vi "ScriptTest.vi"() -> ()   [LabVIEW 2012]
panel:
  out "Variables":string="0: VER = 9\r\n1: HI = 1\r\n2: LO = 0\r\n3: END = 22\r\n4: variable = 13\r\n5: count1 = 4\r\n6: var = 2\r\n7: array_SIZE = 10\r\n8: array_0 = 0\r\n9: array_1 = 0\r\n10: array_2 = 0\r\n11: array_3 = 3\r\n12: array_4 = 0\r\n13: array_5 = 1\r\n14: array_6 = 0\r\n15: array_7 = 0\r\n16: array_8 = 0\r\n17: array_9 = 0\r\n18: count0 = 2\r\n"
  out "Array":bool[](array[boolean])=[TRUE, TRUE, TRUE, FALSE, TRUE, TRUE, TRUE]
  out "Received replies":string[](array[string])=["0\n1\n2\n4", "1\n1\n1\n1\n1", "1\n50\n1\n1", "1\n0\n200\n231\n247\n1\n200\n226", "10\n1\n0\n3\n3\n3\n0", "[1,115]  start script\n [5,61,0,18,0,0]  \n [5,61,202,13,0,1]  \n [3,87,3,232]  \n [5,61,202,13,0,0]  \n [3,87,3,232]  \n [5,43,0,18,0,1]  \n [8,73,60,255,18,0,2,0,5]  \n [1,101]  \n [1,69]  61,0,18,0,0,61,202,13,0,1,87,3,232,61,202,13,0,0,87,3,232,43,0,18,0,1,73,60,255,18,0,2,0,5,101,end script\n0\n1\n1000\n0\n1000\n1\n5\n1\n1000\n0\n1000\n2\n34\nDone", "2\n [1,115]  start script\n [5,61,202,13,0,0]  \n [8,33,6,255,4,0,13,0,2]  \n [3,119,0,1]  \n [5,61,202,13,0,1]  \n [1,101]  \n [1,69]  61,202,13,0,0,33,6,255,4,0,13,0,2,119,0,1,61,202,13,0,1,101,end script\n0\n13\n1\n1\nDone"]
  in  "Expected replies":string[](array[string])=["0\n1\n2\n4", "1\n1\n1\n1\n1", "1\n50\n1\n1", "1\r\n0\r\n200\r\n226\r\n241\r\n1\r\n200\r\n231\r", "10\n1\n0\n3\n3\n3\n0", "[1,115]  start script\n [5,61,0,18,0,0]  \n [5,61,202,13,0,1]  \n [3,87,3,232]  \n [5,61,202,13,0,0]  \n [3,87,3,232]  \n [5,43,0,18,0,1]  \n [8,73,60,255,18,0,2,0,5]  \n [1,101]  \n [1,69]  61,0,18,0,0,61,202,13,0,1,87,3,232,61,202,13,0,0,87,3,232,43,0,18,0,1,73,60,255,18,0,2,0,5,101,end script\n0\n1\n1000\n0\n1000\n1\n5\n1\n1000\n0\n1000\n2\n34\nDone", "2\n [1,115]  start script\n [5,61,202,13,0,0]  \n [8,33,6,255,4,0,13,0,2]  \n [3,119,0,1]  \n [5,61,202,13,0,1]  \n [1,101]  \n [1,69]  61,202,13,0,0,33,6,255,4,0,13,0,2,119,0,1,61,202,13,0,1,101,end script\n0\n13\n1\n1\nDone"]
  in  "Test codes":string[](array[string])=["SET count1,0\nADD count1,1\nADD count1,count1\nADD count1,count1\n", "SET var,1\nSET DIO[0],1\nSET DIO[2],var\nSET DIO[var],var\nSET DIO[30],1\n", "SET var,1\nSET PWM[0],50\nSET PWM[2],var\nSET PWM[var],var\n", "SET var,1\nSET TMR[1],0\nWAIT 0.2\nGET TMR[1]\nGET TMR[var]\nSET TMR[var],var\nWAIT 0.2\nGET TMR[var]", "SET array_SIZE,10\nSET array[5],1\nGET array[0]\nSET var,3\nSET array[var],var\nGET array[var]\nGET array[10]\n", "SCRIPT\ncount0=0\n//while0 for 2 iterations\nwhileLand0:\nDIO[13] = 1\nWAIT 1.000000\nDIO[13] = 0\nWAIT 1.000000\n//end while0 \ncount0+=1\nIF (count0 < 2) GOTO whileLand0\nend\nENDSCRIPT\nRUN&WAIT 0", "SYSTEM var,2,5\nSCRIPT\nDIO[13] = 0\nSYSTEM variable,13,2\nWAITµs 1.000000\nDIO[13] = 1\nend\nENDSCRIPT\nRUN&WAIT 0"]
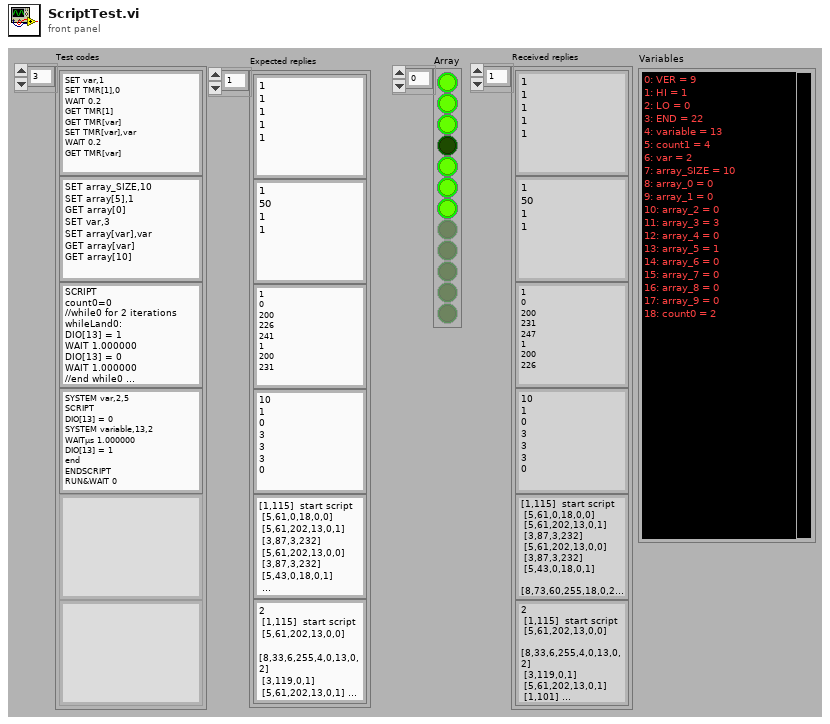
[diagram p1: front panel]
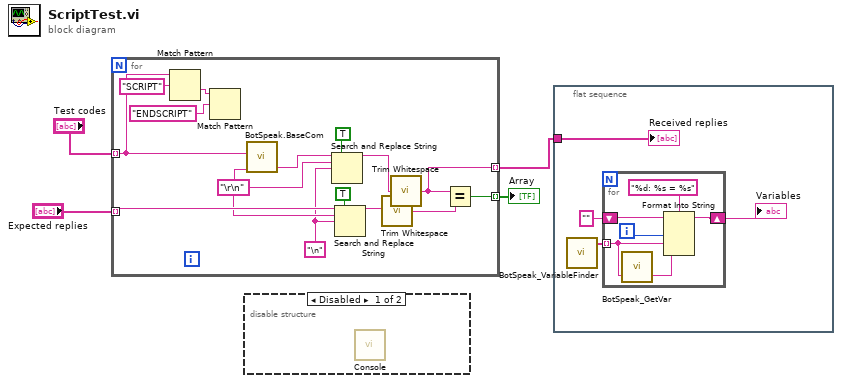
[diagram p0: block diagram]
diagram:
  n1 = for {
    tunnel: "Test codes" -> [w8] mode=indexing
    tunnel: [w17] -> w3 mode=indexing
    tunnel: "Expected replies" -> [w15] mode=indexing
    tunnel: [w19] -> w1 mode=indexing
    w9 = "\n" ("Termination")
    w10 = "\r\n" ("Termination")
    n2 = Match Pattern(string=w8, regular expression="SCRIPT") -> (after substring=w6:string)  [unwired: 1 in, 3 out]
    n3 = Match Pattern(string=w6, regular expression="ENDSCRIPT") -> ()  [unwired: 1 in, 4 out]
    n4 = call <userlib>:"BotSpeak.BaseCom.vi"("Termination"=w10, "command"=w8) -> ("response"=w12:string)  [unwired: 3 in, 1 out]
    n5 = Search and Replace String(replace all?=TRUE ("replace all? (F)"), input string=w12, search string=w10, replace string=w9) -> (result string=w11:string)  [unwired: 4 in, 3 out]
    n6 = Search and Replace String(replace all?=TRUE ("replace all? (F)"), input string=w15, search string=w10, replace string=w9) -> (result string=w16:string)  [unwired: 4 in, 3 out]
    n7 = call <vilib>:"Trim Whitespace.vi"("string"=w16) -> ("trimmed string"=w18:string)  [unwired: 1 in]
    n8 = call <vilib>:"Trim Whitespace.vi"("string"=w11) -> ("trimmed string"=w17:string)  [unwired: 1 in]
    n9 = Equal?(x=w17, y=w18) -> (x = y?=w19:bool)
  }
  "Array" <- w1
  n10 = disable-structure shown="Disabled" {
    frame Disabled {
      n11 = call <userlib>:"Console.vi"() -> ()  [unwired: 4 in, 1 out]
    }
    frame Enabled {
    }
  }
  n12 = flat-sequence {
    tunnel: w3 -> [w23]
    frame #0 {
      n13 = call <userlib>:"BotSpeak_VariableFinder.vi"() -> ("Variables"=w22:string[])  [unwired: 3 in, 1 out]
      n14 = for {
        tunnel: w22 -> [w25] mode=indexing
        shift-right: [w27] -> w20
        shift-left: "" -> [w26]
        i -> [w28]
        n15 = call <userlib>:"BotSpeak_GetVar.vi"("Variable In"=w25) -> ("value"=w24:string)  [unwired: 1 in, 1 out]
        n16 = Format Into String(format string="%d: %s = %s", initial string=w26, w28, w25, w24) -> (resulting string=w27:string)  [unwired: 1 in, 1 out]
      }
      "Variables" <- w20
      "Received replies" <- w23
    }
  }
